vi "SelectClassIcon.vi"() -> ()   [LabVIEW 2020]
uses:
  <vilib>/Utility/miscctls.llb/LVBoundsTypeDef.ctl
  <resource>/Framework/Providers/Open_GDS/ClassProviders/Common/CommonVIs/CommonVIs_ClassIconSelection_Action.ctl
  c84afe10-fc65-4d8b-b200-0de5f07e0a9c.vi
  8146e3c4-7363-43e9-93da-efe32bb20ee4.vi
panel:
  out "IconSelected":string
  in  "error in (no error)":errorcluster
  out "IconSelection":picture
  out "Icon":picture
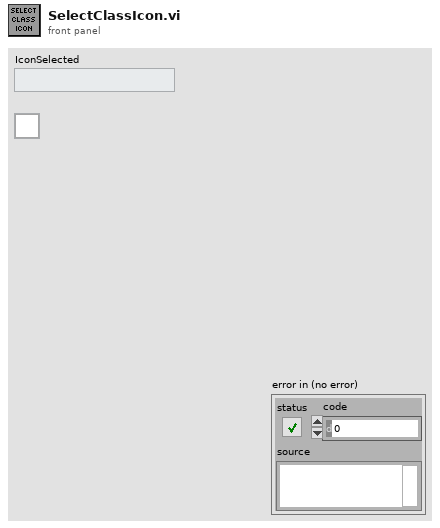
[diagram p1: front panel]
types:
  T1 = typedef "CommonVIs_ClassIconSelection_Action.ctl" = enum16{"All", "Non Interface", "Only Interface"}
  T2 = typedef "LVBoundsTypeDef.ctl" = cluster{"Width":u32, "Height":u32}
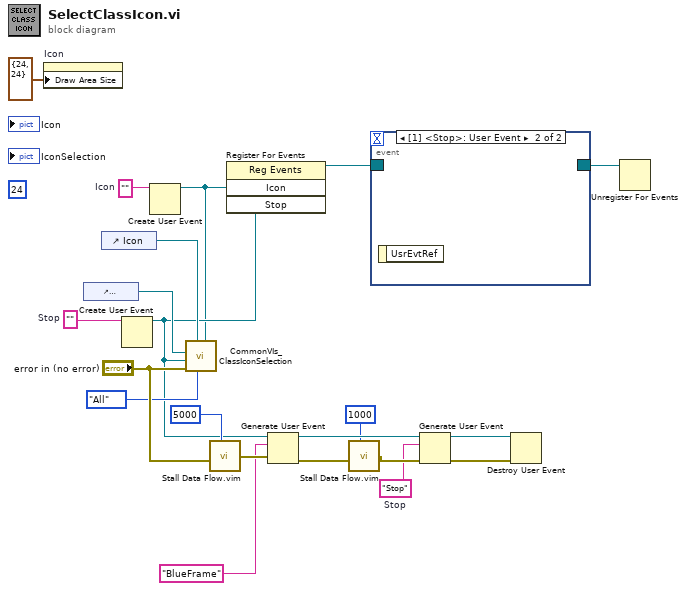
[diagram p0: block diagram]
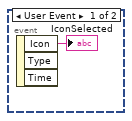
[diagram p2: hidden frame]
diagram:
  w6 = ""  # Icon
  w9 = "Stop"  # Stop
  w15 = ""  # Stop
  (unwired) u32 24 ("Height")
  n1 = property on="Icon" class="Pict"("Draw Area Size"=T2 {"Width"=24, "Height"=24}) -> ()  [unwired: 2 in, 2 out]
  n2 = control-ref of="IconSelection"() -> (w19:refnum<vi>)
  n3 = control-ref of="Icon"() -> (w20:refnum<vi>)
  n4 = Create User Event(user event datatype=w15) -> (user event=w4:refnum<user-event>)  [unwired: 1 in, 1 out]
  n5 = Create User Event(user event datatype=w6) -> (user event=w3:refnum<user-event>)  [unwired: 1 in, 1 out]
  n6 = call <resource>:"CommonVIs_ClassIconSelection.vi"("IconSelected"=w3, "IconsToShow(All)"=CommonVIs_ClassIconSelection_Action."All", "Icon"=w20, "error in (no error)"="error in (no error)", "Messages(Stop or Empty string will stop this VI)"=w4, "IconSelection"=w19) -> ()  [unwired: 6 in]
  n7 = call "Stall Data Flow.vim"("value in"="error in (no error)", "milliseconds to wait"=u32 5000) -> ("value out"=w17:errorcluster)  [unwired: 1 out]
  n8 = register-events(w3, w4) -> (reference out=w5:refnum<event-registration>)  [unwired: 2 in, 1 out]
  n9 = Generate User Event(user event=w4, event data cluster="BlueFrame", error in=w17) -> (user event out=w12:refnum<user-event>, error out=w14:errorcluster)  [unwired: 1 in]
  n10 = call "Stall Data Flow.vim"("value in"=w14, "milliseconds to wait"=u32 1000) -> ("value out"=w13:errorcluster)  [unwired: 1 out]
  n11 = event shown="[1] <Stop>: User Event" {
    selector: w5 -> [_ _]
    dyn-events: [_ _] -> w2
    timeout: _ -> [_ _]
    event User Event {
      n12 = event-data() -> ("Icon"=→"IconSelected":string)  [unwired: 1 in, 2 out]
    }
    event User Event {
      n13 = event-data() -> ()  [unwired: 1 in, 1 out]
    }
  }
  n14 = Generate User Event(user event=w12, event data cluster=w9, error in=w13) -> (user event out=w11:refnum<user-event>, error out=w10:errorcluster)  [unwired: 1 in]
  n15 = Destroy User Event(user event=w11, error in=w10) -> ()  [unwired: 1 out]
  n16 = Unregister For Events(event registration refnum=w2) -> ()  [unwired: 1 in, 1 out]
